vi "Configure Frequency Sweep.vi"(4 "Stop  Frequency  (1000.0 Hz)":dbl=1000.0 format="%#.6g", 6 "Start Frequency (100.0 Hz)":dbl=100.0 format="%#.6g", 7 "Enable Frequency Sweep (T:Enable)":bool=TRUE, 8 "error in (no error)":errorcluster, 9 "Sweep Time (1.00 s)":dbl=1.0 format="%#.6g", 10 "Sweep Spacing (0: Linear)":u16(ring) items=["Linear", "Log"], 11 "VISA resource name":refnum<visa-resource-name>) -> (0 "error out":errorcluster, 3 "VISA resource name out":refnum<visa-resource-name>)   [LabVIEW 2012, in "Novatech 409b.lvlib"]
doc: "Configures and enables a frequency sweep. In the frequency sweep mode, the function generator steps from the start frequency to the stop frequency at a sweep rate."
uses:
  <instrlib>/Novatech 409b/Novatech 409b.lvlib
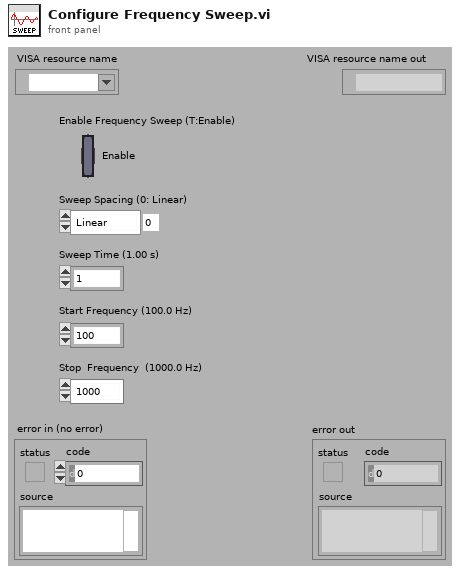
[diagram p1: front panel]
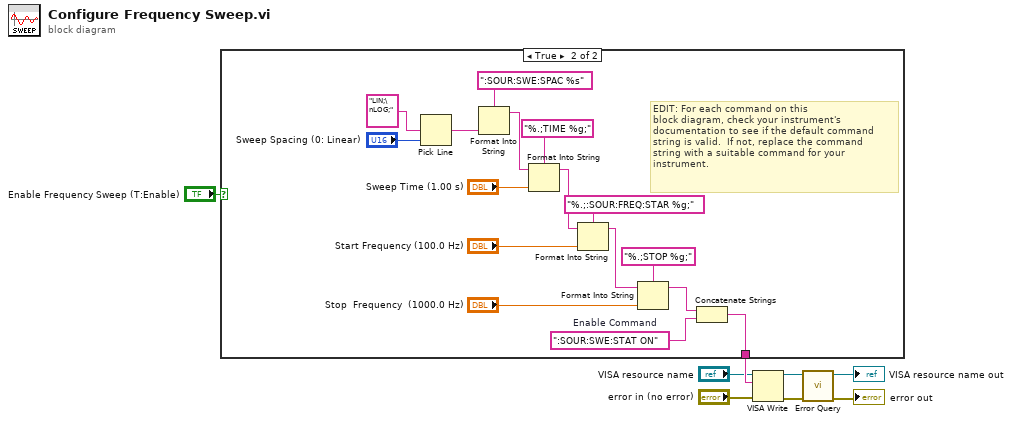
[diagram p0: block diagram]
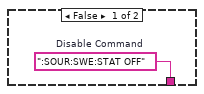
[diagram p2: hidden frame]
diagram:
  n1 = case shown="True" "Enable Frequency Sweep (T:Enable)" {
    tunnel: [w9 w12] -> w7
    frame False {
      w9 = ":SOUR:SWE:STAT OFF"  # Disable Command
    }
    frame True {
      w10 = ":SOUR:SWE:STAT ON"  # Enable Command
      # "EDIT: For each command on this\nblock diagram, check your instrument's\ndocumentation to see if the default command\nstring is valid.  If not, replace the command\nstring with a suitable command for your\ninstrument."
      n2 = Pick Line(multi-line string="LIN;\nLOG;", line index="Sweep Spacing (0: Linear)") -> (output string=w16:string)  [unwired: 1 in]
      n3 = Format Into String(format string=":SOUR:SWE:SPAC %s", w16) -> (resulting string=w15:string)  [unwired: 2 in, 1 out]
      n4 = Format Into String(format string="%.;TIME %g;", initial string=w15, "Sweep Time (1.00 s)") -> (resulting string=w22:string)  [unwired: 1 in, 1 out]
      n5 = Format Into String(format string="%.;:SOUR:FREQ:STAR %g;", initial string=w22, "Start Frequency (100.0 Hz)") -> (resulting string=w19:string)  [unwired: 1 in, 1 out]
      n6 = Format Into String(format string="%.;STOP %g;", initial string=w19, "Stop  Frequency  (1000.0 Hz)") -> (resulting string=w11:string)  [unwired: 1 in, 1 out]
      n7 = Concatenate Strings(w11, w10) -> (w12:string)
    }
  }
  n8 = VISA Write(VISA resource name="VISA resource name", write buffer=w7, error in (no error)="error in (no error)") -> (VISA resource name out=w5:refnum<visa-resource-name>, error out=w3:errorcluster)  [unwired: 1 out]
  n9 = call <instrlib>:"Error Query.vi"("error in (no error)"=w3, "VISA resource name"=w5) -> ("error out"=→"error out":errorcluster, "VISA resource name out"=→"VISA resource name out":refnum<visa-resource-name>)  [unwired: 6 in, 2 out]
